vi "Open Accelerometer SPI.vi"(6 "Clock Rate in kHz":u16=1000, 7 "Chip Select":u32, 8 "error in (no error)":errorcluster, 11 "Device":T2="USB0::0x3923::0x7166::01879089::RAW") -> (0 "error out":errorcluster, 3 "Accelerometer":T1, 4 "good":bool, 5 "whoami":u8)   [LabVIEW 2013]
doc: "Use this template to build a VI to use as a subVI."
uses:
  <vilib>/ni845x/ni845x.llb/ni845xControl.ctl
  AccelerometerSPI.ctl
  <vilib>/ni845x/ni845x.llb/ni845xSpiConfiguration.ctl
  9250registers.ctl
  <resource>/objmgr/NI845x.rc
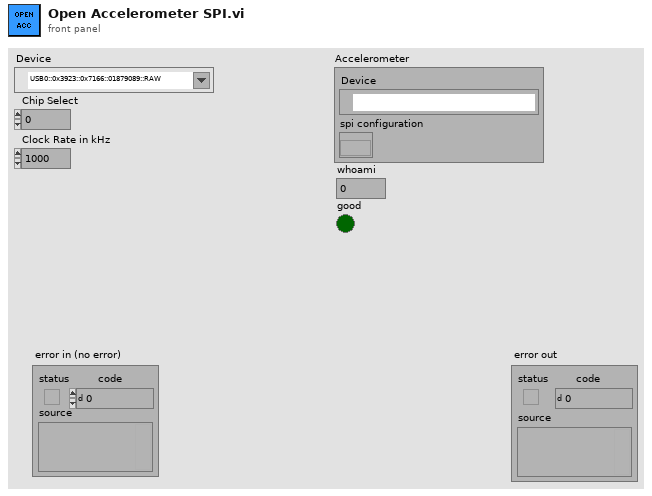
[diagram p1: front panel]
types:
  T1 = typedef "AccelerometerSPI.ctl" = cluster{"Device":T2, "spi configuration":T3}
  T2 = typedef "ni845xControl.ctl" = refnum<k21>
  T3 = typedef "ni845xSpiConfiguration.ctl" = refnum<k20>
  T4 = typedef "9250registers.ctl" = u8
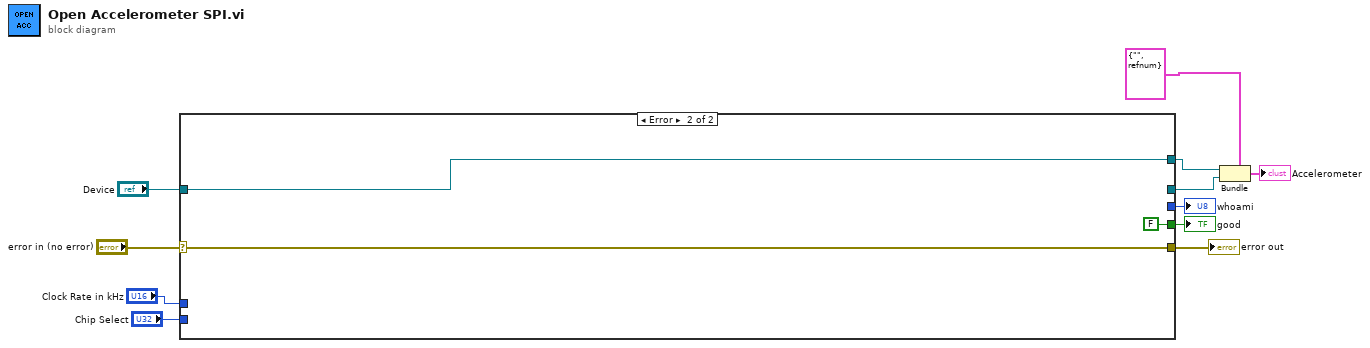
[diagram p0: block diagram]
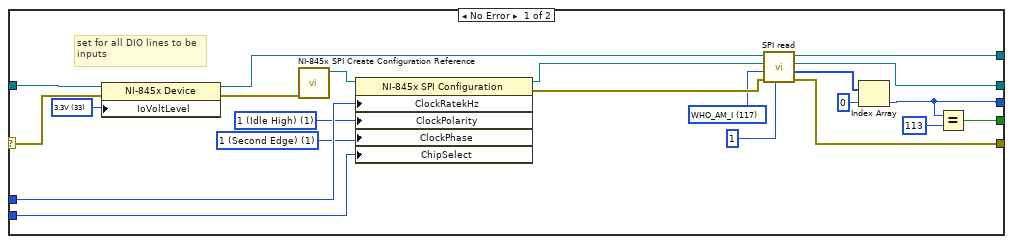
[diagram p2: hidden frame]
diagram:
  n1 = case shown="Error" "error in (no error)" {
    selector: "error in (no error)" -> [w31 w36]
    tunnel: [w18 w36] -> w10
    tunnel: "Device" -> [w32 w35]
    tunnel: [w17 _] -> w7
    tunnel: [w24 w35] -> w8
    tunnel: "Clock Rate in kHz" -> [w28 _]
    tunnel: "Chip Select" -> [w25 _]
    tunnel: [w14 _] -> w2
    tunnel: [w12 FALSE] -> w1
    frame No Error {
      w20 = T4 117 items=["SELF_TEST_X_GYRO"=0, "SELF_TEST_Y_GYRO"=1, "SELF_TEST_Z_GYRO"=2, "SELF_TEST_X_ACCEL"=13, "SELF_TEST_Y_ACCEL"=14, "SELF_TEST_Z_ACCEL"=15, "XG_OFFSET"=19, "YG_OFFSET"=21, "ZG_OFFSET"=23, "SMPLRT_DIV"=25, "CONFIG"=26, "GYRO_CONFIG"=27, "ACCEL_CONFIG"=28, "ACCEL_CONFIG2"=29, "FIFO_EN"=35, "I2C_MST_CTRL"=36, "I2C_SLV0_ADDR"=37, "I2C_SLV0_REG"=38, "I2C_SLV0_CTRL"=39, "I2C_MST_STATUS"=54, "INT_ENABLE"=56, "INT_STATUS"=58, "ACCEL_XOUT"=59, "ACCEL_YOUT"=61, "ACCEL_ZOUT"=63, "TEMP_OUT"=65, "GYRO_XOUT"=67, "GYRO_YOUT"=69, "GYRO_ZOUT"=71, "EXT_SENS_DATA_00"=73, "I2C_SLV0_D0"=99, "USER_CTRL"=106, "PWR_MGMT_1"=107, "PWR_MGMT_2"=108, "WHO_AM_I"=117, "XA_OFFSET"=119, "YA_OFFSET"=122, "ZA_OFFSET"=125] ("Address")
      w26 = 1 items=["0 (First Edge)", "1 (Second Edge)"] ("Clock Phase")
      w27 = 1 items=["0 (Idle Low)", "1 (Idle High)"] ("Clock Polarity")
      w33 = 33 items=["3.3V"=33, "2.5V"=25, "1.8V"=18, "1.5V"=15, "1.2V"=12] ("I/O Voltage Level")
      # "set for all DIO lines to be\ninputs"
      n2 = property on="Property Node" class="NI-845x Device"(reference=w32, error in=w31, "IoVoltLevel"=w33) -> (reference out=w23:T2, error out=w30:errorcluster)
      n3 = call <vilib>:"NI-845x SPI Create Configuration Reference.vi"("error in (no error)"=w30) -> ("spi configuration"=w29:T3)  [unwired: 9 in, 1 out]
      n4 = property class="NI-845x SPI Configuration"(reference=w29, "ClockRatekHz"=w28, "ClockPolarity"=w27, "ClockPhase"=w26, "ChipSelect"=w25) -> (reference out=w22:T3, error out=w21:errorcluster)  [unwired: 1 in]
      n5 = call "SPI read.vi"("Number of bytes"=1, "error in (no error)"=w21, "Address"=w20, "spi configuration in"=w22, "Device ref in"=w23) -> ("error out"=w18:errorcluster, "read data"=w16:u8[], "spi configuration out"=w17:T3, "Device ref out"=w24:T2)  [unwired: 3 in]
      n6 = Index Array(array=w16, index=0) -> (element=w14:u8)
      n7 = Equal?(x=w14, y=u8 113) -> (x = y?=w12:bool)
    }
    frame Error {
    }
  }
  "error out" <- w10
  "whoami" <- w2
  "good" <- w1
  n8 = Bundle(cluster=T1 {"Device"="", "spi configuration"=refnum} ("Accelerometer"), "Device"=w8, "spi configuration"=w7) -> (→"Accelerometer":T1)
